vi "Run.vi"(8 "error in (no error)":errorcluster, 11 "GSdevice in":refnum<class "GSdevice.lvclass">) -> (0 "error out":errorcluster, 3 "GSdevice out":refnum<class "GSdevice.lvclass">)   [LabVIEW 2018, in "GSdevice.lvclass"]
uses:
  GSdevice.lvclass
  GSdevice.lvclass/GSdevice.ctl
  Device/Device.lvclass
  StateMachine/State Machine.lvclass
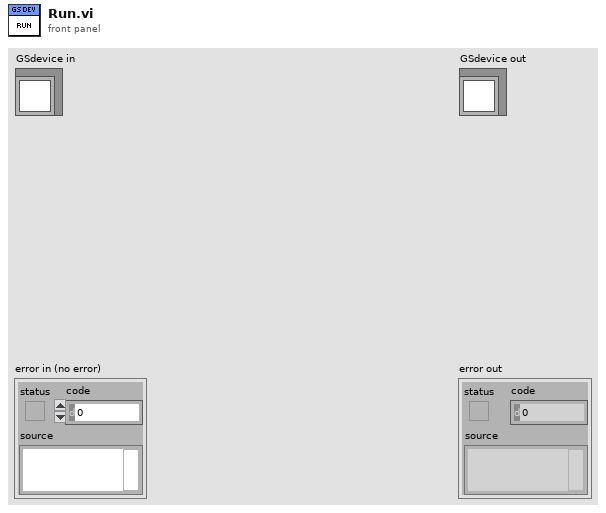
[diagram p1: front panel]
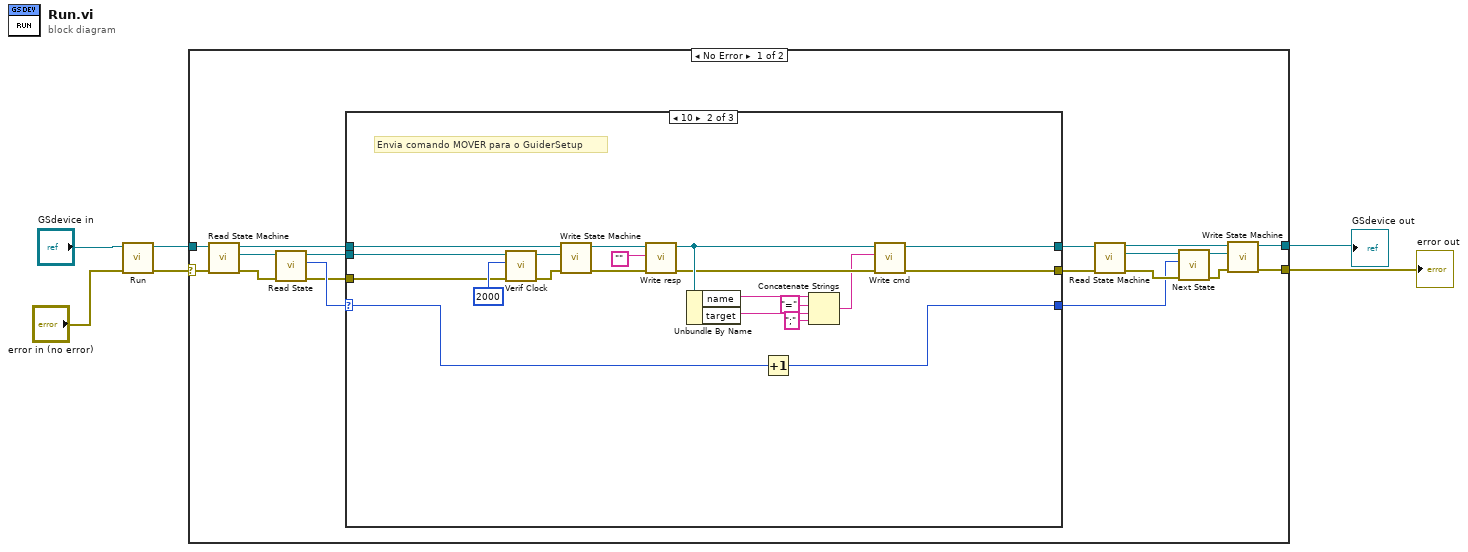
[diagram p0: block diagram]
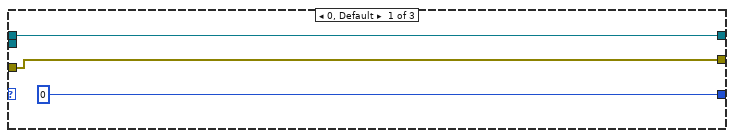
[diagram p2: hidden frame]
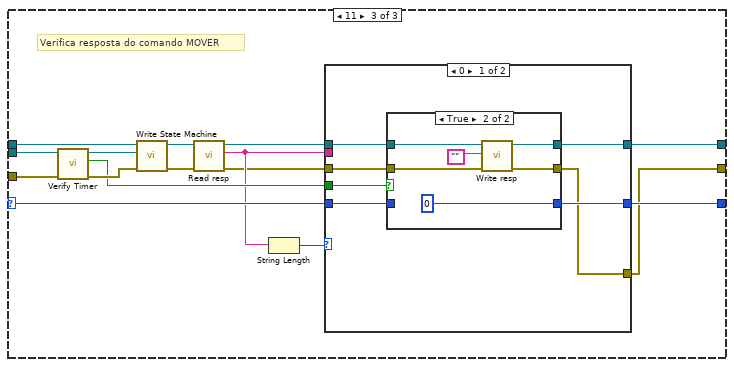
[diagram p3: hidden frame]
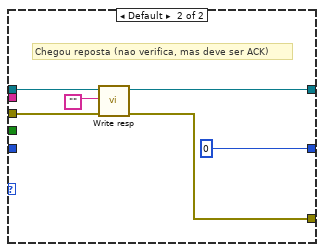
[diagram p5: hidden frame]
diagram:
  n1 = call-parent "Run.vi"("error in (no error)"="error in (no error)", "Device in"="GSdevice in") -> ("error out"=w3:errorcluster, "Device out"=w4:refnum<class "GSdevice.lvclass">)  [unwired: 8 in]
  n2 = case shown="No Error" w3 {
    selector: w3 -> [w23 w87]
    tunnel: [w15 w87] -> w1
    tunnel: w4 -> [w24 w86]
    tunnel: [w14 w86] -> w2
    frame No Error {
      n3 = call-dynamic "Read State Machine.vi"("error in (no error)"=w23, "Device in"=w24) -> ("error out"=w21:errorcluster, "State Machine.lvclass"=w22:refnum<class "State Machine.lvclass">, "Device out"=w12:refnum<class "GSdevice.lvclass">)  [unwired: 7 in]
      n4 = call-dynamic "Read State.vi"("error in (no error)"=w21, "State Machine in"=w22) -> ("error out"=w11:errorcluster, "State"=w13:i32, "State Machine out"=w7:refnum<class "State Machine.lvclass">)  [unwired: 7 in]
      n5 = case shown="10" w13 {
        selector: w13 -> [_ w37 w53]
        tunnel: w12 -> [w26 w47 w58]
        tunnel: w11 -> [w25 w30 w56]
        tunnel: [w25 w36 w48] -> w10
        tunnel: [w26 w35 w62] -> w9
        tunnel: [0 ("State") w34 w61] -> w8
        tunnel: w7 -> [_ w32 w60]
        frame 0, Default {
        }
        frame 10 {
          # "Envia comando MOVER para o GuiderSetup"
          n6 = call-dynamic "Verif Clock.vi"("error in (no error)"=w30, "period (ms)"=u32 2000 ("period"), "State Machine in"=w32) -> ("error out"=w29:errorcluster, "State Machine out"=w31:refnum<class "State Machine.lvclass">)  [unwired: 6 in, 1 out]
          n7 = call-dynamic "Write State Machine.vi"("error in (no error)"=w29, "State Machine.lvclass"=w31, "Device in"=w47) -> ("error out"=w45:errorcluster, "Device out"=w46:refnum<class "GSdevice.lvclass">)  [unwired: 7 in]
          n8 = call-dynamic "Write resp.vi"("error in (no error)"=w45, "resp"="", "Device in"=w46) -> ("error out"=w39:errorcluster, "Device out"=w40:refnum<class "GSdevice.lvclass">)  [unwired: 7 in]
          n9 = Unbundle By Name(w40) -> ("name"=w43:string, "target"=w41:string)
          n10 = Increment(x=w37) -> (x+1=w34:i32)
          n11 = Concatenate Strings(w43, "=" ("string"), w41, ";" ("string")) -> (w38:string)
          n12 = call-dynamic "Write cmd.vi"("error in (no error)"=w39, "cmd"=w38, "Device in"=w40) -> ("error out"=w36:errorcluster, "Device out"=w35:refnum<class "GSdevice.lvclass">)  [unwired: 7 in]
        }
        frame 11 {
          # "Verifica resposta do comando MOVER"
          n13 = call "Verify Timer.vi"("error in (no error)"=w56, "State Machine in"=w60) -> ("error out"=w57:errorcluster, "timeout"=w52:bool, "State Machine out"=w59:refnum<class "State Machine.lvclass">)  [unwired: 7 in]
          n14 = call-dynamic "Write State Machine.vi"("error in (no error)"=w57, "State Machine.lvclass"=w59, "Device in"=w58) -> ("error out"=w54:errorcluster, "Device out"=w55:refnum<class "GSdevice.lvclass">)  [unwired: 7 in]
          n15 = call-dynamic "Read resp.vi"("error in (no error)"=w54, "Device in"=w55) -> ("error out"=w49:errorcluster, "resp"=w50:string, "Device out"=w63:refnum<class "GSdevice.lvclass">)  [unwired: 7 in]
          n16 = String Length(string=w50) -> (length=w51:i32)
          n17 = case shown="0" w51 {
            tunnel: w63 -> [w67 w85]
            tunnel: [w66 w81] -> w62
            tunnel: [w69 0 ("State")] -> w61
            tunnel: w53 -> [w70 _]
            tunnel: w52 -> [w68 _]
            tunnel: w50 -> [_ _]
            tunnel: w49 -> [w65 w82]
            tunnel: [w64 w80] -> w48
            frame 0 {
              n18 = case shown="True" w68 {
                tunnel: w70 -> [w73 _]
                tunnel: [w73 0 ("State")] -> w69
                tunnel: [w71 w76] -> w66
                tunnel: w67 -> [w71 w77]
                tunnel: w65 -> [w72 w75]
                tunnel: [w72 w74] -> w64
                frame False {
                }
                frame True {
                  n19 = call-dynamic "Write resp.vi"("error in (no error)"=w75, "resp"="", "Device in"=w77) -> ("error out"=w74:errorcluster, "Device out"=w76:refnum<class "GSdevice.lvclass">)  [unwired: 7 in]
                }
              }
            }
            frame Default {
              # "Chegou reposta (nao verifica, mas deve ser ACK)"
              n20 = call-dynamic "Write resp.vi"("error in (no error)"=w82, "resp"="", "Device in"=w85) -> ("error out"=w80:errorcluster, "Device out"=w81:refnum<class "GSdevice.lvclass">)  [unwired: 7 in]
            }
          }
        }
      }
      n21 = call-dynamic "Read State Machine.vi"("error in (no error)"=w10, "Device in"=w9) -> ("error out"=w17:errorcluster, "State Machine.lvclass"=w19:refnum<class "State Machine.lvclass">, "Device out"=w18:refnum<class "GSdevice.lvclass">)  [unwired: 7 in]
      n22 = call "Next State.vi"("error in (no error)"=w17, "New_State"=w8, "State Machine in"=w19) -> ("error out"=w16:errorcluster, "State Machine out"=w20:refnum<class "State Machine.lvclass">)  [unwired: 7 in]
      n23 = call-dynamic "Write State Machine.vi"("error in (no error)"=w16, "State Machine.lvclass"=w20, "Device in"=w18) -> ("error out"=w15:errorcluster, "Device out"=w14:refnum<class "GSdevice.lvclass">)  [unwired: 7 in]
    }
    frame Error {
    }
  }
  "error out" <- w1
  "GSdevice out" <- w2
